vi "Split String to Array.vi"(1 "搜索字符串/字符(-)":string="-", 2 "字符串":string) -> (0 "字符串数组":string[](array[string]))   [LabVIEW 2011]
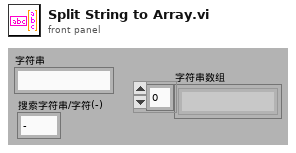
[diagram p1: front panel]
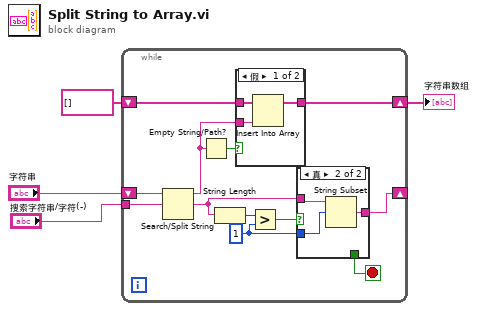
[diagram p0: block diagram]
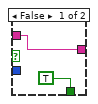
[diagram p2: hidden frame]
diagram:
  n1 = while {
    shift-right: [w7] -> _
    shift-left: "字符串" -> [w16]
    shift-right: [w12] -> w3
    shift-left: string[] [] ("项名称") -> [w14]
    tunnel: "搜索字符串/字符(-)" -> [w5]
    stop <- w6 stop-if-true
    w8 = 1 ("y")
    n2 = Search/Split String(string=w16, search string/char (-)=w5) -> (substring before match=w13:string, match + rest of string=w9:string)  [unwired: 2 out]
    n3 = Empty String/Path?(string/path=w13) -> (empty?=w15:bool)
    n4 = String Length(string=w9) -> (length=w11:i32)
    n5 = case shown="假" w15 {
      tunnel: w14 -> [w24 w25]
      tunnel: w13 -> [w23 _]
      tunnel: [w22 w25] -> w12
      frame False {
        n6 = Insert Into Array(array=w24, new element=w23) -> (w22:string[])  [unwired: 1 in]
      }
      frame True {
      }
    }
    n7 = Greater?(x=w11, y=w8) -> (0:w10:bool)
    n8 = case shown="真" w10 {
      tunnel: w9 -> [w18 w21]
      tunnel: w8 -> [_ w20]
      tunnel: [w18 w19] -> w7
      tunnel: [TRUE _] -> w6
      frame False {
      }
      frame True {
        n9 = String Subset(string=w21, offset (0)=w20) -> (substring=w19:string)  [unwired: 1 out]
      }
    }
  }
  "字符串数组" <- w3
